vi "BuildConstructor.vi"(7 "PythonConverter_BD in":refnum<class "PyConvBD.lvclass">, 8 "error in":errorcluster, 11 "Function in":refnum<class "CompoundArithmetic.lvclass">) -> (0 "error out":errorcluster, 3 "Function out":refnum<class "CompoundArithmetic.lvclass">, 4 "constructor":string, 5 "PythonConverter_BD out":refnum<class "PyConvBD.lvclass">)   [LabVIEW 2014, in "CompoundArithmetic.lvclass"]
uses:
  CompoundArithmetic.lvclass
  Python/PythonConverter_BD/PyConvBD.lvclass
  Python/Parsing/Classes/PythonFunction/PythonFunction.lvclass/PythonFunction.ctl
  CompoundArithmetic.lvclass/CompoundArithmetic.ctl
  Python/Parsing/Classes/PythonFunction/PythonFunction.lvclass
  GrowableFunction/GrowableFunction.lvclass
  Python/Parsing/Python Functions.lvlib
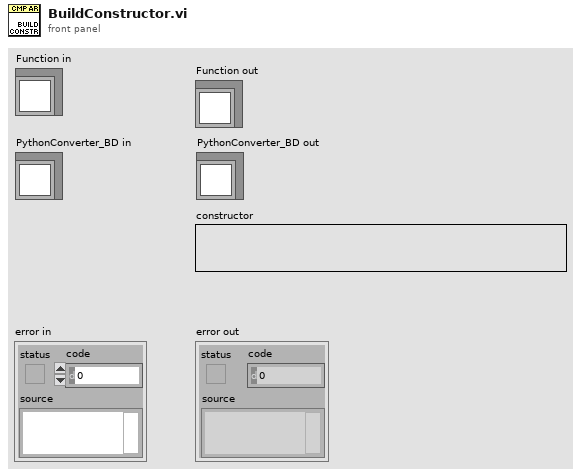
[diagram p1: front panel]
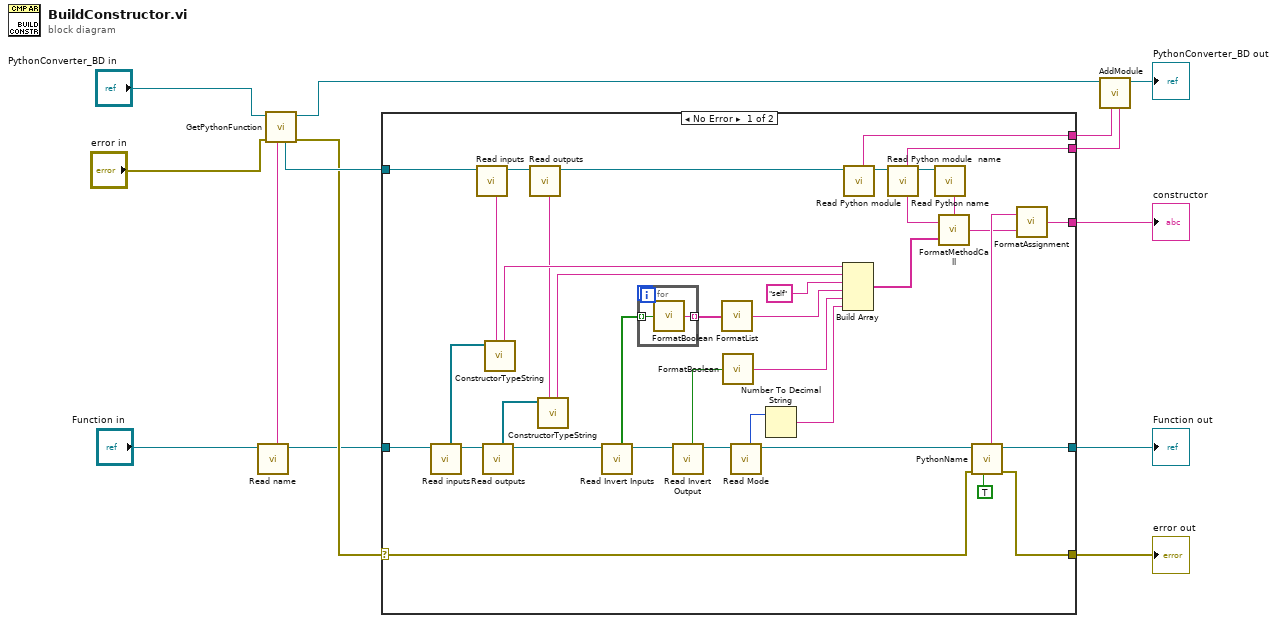
[diagram p0: block diagram]
diagram:
  n1 = call-dynamic "Read name.vi"("Node in"="Function in") -> ("Node out"=w8:refnum<class "CompoundArithmetic.lvclass">, "name"=w9:string)  [unwired: 7 in]
  n2 = call "GetPythonFunction.vi"("function name"=w9, "error in"="error in", "PythonConverter_BD in"="PythonConverter_BD in") -> ("error out"=w13:errorcluster, "PythonConverter_BD out"=w12:refnum<class "PyConvBD.lvclass">, "Python function"=w14:refnum<class "PythonFunction.lvclass">)  [unwired: 4 in]
  n3 = case shown="No Error" w13 {
    selector: w13 -> [w17 w54]
    tunnel: [w16 w54] -> w4
    tunnel: [w23 _] -> w1
    tunnel: w14 -> [w44 _]
    tunnel: [w49 _] -> w11
    tunnel: [w28 _] -> w10
    tunnel: w8 -> [w43 w53]
    tunnel: [w24 w53] -> w6
    frame No Error {
      n4 = call-dynamic "Read inputs.vi"("Node in"=w43) -> ("Node out"=w41:refnum<class "CompoundArithmetic.lvclass">, "inputs"=w42:refnum<class "Terminal.lvclass">[])  [unwired: 7 in]
      n5 = call "Read inputs.vi"("PythonFunction in"=w44) -> ("PythonFunction out"=w45:refnum<class "PythonFunction.lvclass">, "inputs"=w46:string)  [unwired: 7 in]
      n6 = call-dynamic "Read outputs.vi"("Node in"=w41) -> ("Node out"=w18:refnum<class "CompoundArithmetic.lvclass">, "outputs"=w40:refnum<class "Terminal.lvclass">[])  [unwired: 7 in]
      n7 = call "ConstructorTypeString.vi"("list"=w46, "terminals"=w42) -> ("constructor string"=w50:string)  [unwired: 7 in]
      n8 = call "Read outputs.vi"("PythonFunction in"=w45) -> ("PythonFunction out"=w19:refnum<class "PythonFunction.lvclass">, "outputs"=w47:string)  [unwired: 7 in]
      n9 = call "ConstructorTypeString.vi"("list"=w47, "terminals"=w40) -> ("constructor string"=w21:string)  [unwired: 7 in]
      n10 = call "Read Invert Inputs.vi"("CompoundArithmetic in"=w18) -> ("CompoundArithmetic out"=w37:refnum<class "CompoundArithmetic.lvclass">, "Invert Inputs"=w35:bool[])  [unwired: 7 in]
      n11 = for {
        tunnel: w35 -> [w52] mode=indexing
        tunnel: [w51] -> w34 mode=indexing
        n12 = call "FormatBoolean.vi"("value"=w52) -> ("python object"=w51:string)
      }
      n13 = call "Read Invert Output.vi"("CompoundArithmetic in"=w37) -> ("CompoundArithmetic out"=w38:refnum<class "CompoundArithmetic.lvclass">, "Invert Output"=w36:bool)  [unwired: 7 in]
      n14 = call "FormatList.vi"("values"=w34) -> ("python object"=w33:string)  [unwired: 1 in]
      n15 = call "FormatBoolean.vi"("value"=w36) -> ("python object"=w32:string)
      n16 = call "Read Mode.vi"("CompoundArithmetic in"=w38) -> ("CompoundArithmetic out"=w25:refnum<class "CompoundArithmetic.lvclass">, "Mode"=w31:u32)  [unwired: 7 in]
      n17 = Number To Decimal String(number=w31) -> (decimal integer string=w30:string)  [unwired: 1 in]
      n18 = Build Array(w50, w21, "self" ("element"), w33, w32, w30) -> (w26:string[])
      n19 = call "Read Python module.vi"("PythonFunction in"=w19) -> ("PythonFunction out"=w48:refnum<class "PythonFunction.lvclass">, "Python module"=w49:string)  [unwired: 7 in]
      n20 = call "Read Python module  name.vi"("PythonFunction in"=w48) -> ("PythonFunction out"=w20:refnum<class "PythonFunction.lvclass">, "Python module  name"=w28:string)  [unwired: 7 in]
      n21 = call "Read Python name.vi"("PythonFunction in"=w20) -> ("Python name"=w27:string)  [unwired: 7 in, 1 out]
      n22 = call "FormatMethodCall.vi"("method"=w27, "parameters"=w26, "object"=w28) -> ("python object"=w22:string)
      n23 = call-dynamic "PythonName.vi"("add self"=TRUE, "error in"=w17, "Node in"=w25) -> ("error out"=w16:errorcluster, "Node out"=w24:refnum<class "CompoundArithmetic.lvclass">, "name"=w29:string)  [unwired: 5 in, 1 out]
      n24 = call "FormatAssignment.vi"("value"=w22, "name"=w29) -> ("python assignment"=w23:string)
    }
    frame Error {
    }
  }
  "error out" <- w4
  "Function out" <- w6
  "constructor" <- w1
  n25 = call "AddModule.vi"("python module name"=w10, "python module"=w11, "PythonConverter_BD in"=w12) -> ("PythonConverter_BD out"=→"PythonConverter_BD out":refnum<class "PyConvBD.lvclass">)  [unwired: 5 in, 1 out]
